vi "Configure_single_acquisition.vi"(8 "error in (no error)":errorcluster, 11 "Initialize_card in":refnum<class "Initialize_card.lvclass">) -> (0 "error out":errorcluster, 3 "Initialize_card out":refnum<class "Initialize_card.lvclass">)   [LabVIEW 2015, in "Initialize_card.lvclass"]
uses:
  Initialize_card.lvclass
panel:
  in  "Extended Options (0)":i32
  in  "Invert Clock (f)":bool
  out "Error Code":i32
  in  "Segment Count (1)":u32=1
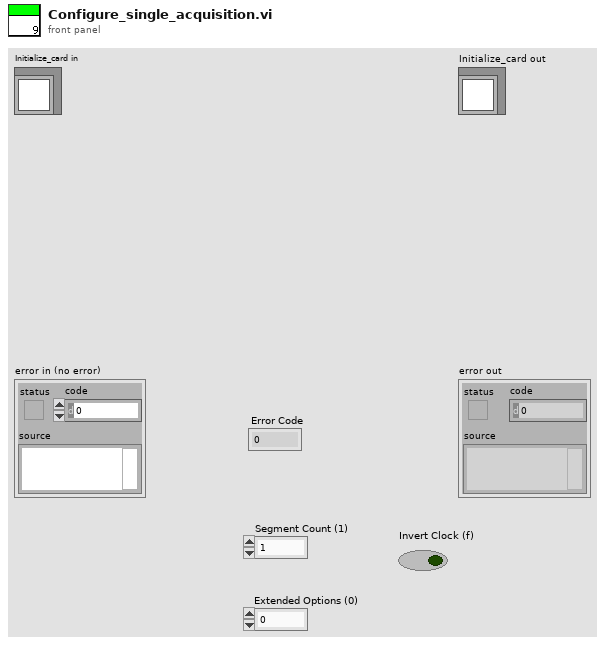
[diagram p1: front panel]
types:
  T1 = cluster{"Sample Rate":dbl, "Clock mode":enum16{"Internal", "External", "Reference"}, "Mode":u16, "Depth":dbl, "Segment Size":dbl, "Trigger Timeout":dbl, "Trigger Holdoff":dbl, "Trigger Delay":dbl}
  T2 = cluster{"Handle":u32, "Sample size":u32, "Resolution":i32, "Offset":i32, "Channels":u32, "Boards":u32}
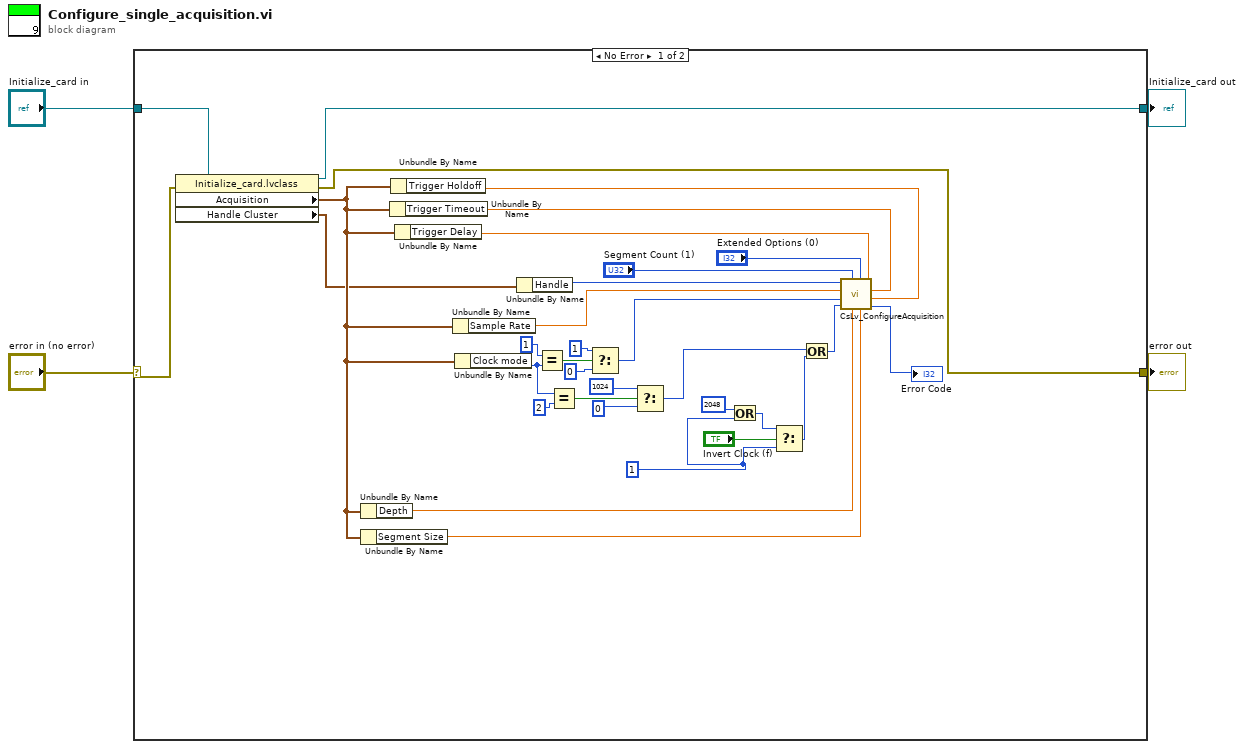
[diagram p0: block diagram]
diagram:
  n1 = case shown="No Error" "error in (no error)" {
    selector: "error in (no error)" -> [w9 w39]
    tunnel: [w8 w39] -> w3
    tunnel: [w10 w38] -> w1
    tunnel: "Initialize_card in" -> [w11 w38]
    frame No Error {
      w6 = 1 ("y")
      n2 = property class="Initialize_card.lvclass"(reference=w11, error in=w9) -> (reference out=w10:refnum<class "Initialize_card.lvclass">, error out=w8:errorcluster, "Acquisition"=w7:T1, "Handle Cluster"=w5:T2)
      n3 = Unbundle By Name(w7) -> ("Depth"=w33:dbl)
      n4 = Unbundle By Name(w7) -> ("Segment Size"=w25:dbl)
      n5 = Unbundle By Name(w7) -> ("Trigger Timeout"=w31:dbl)
      n6 = Unbundle By Name(w7) -> ("Trigger Holdoff"=w30:dbl)
      n7 = Unbundle By Name(w7) -> ("Trigger Delay"=w32:dbl)
      n8 = Unbundle By Name(w7) -> ("Sample Rate"=w34:dbl)
      n9 = Unbundle By Name(w7) -> ("Clock mode"=w19:enum16{"Internal", "External", "Reference"})
      n10 = Unbundle By Name(w5) -> ("Handle"=w37:u32)
      n11 = Equal?(x=1, y=w19) -> (x = y?=w24:bool)
      n12 = Equal?(x=w19, y=2) -> (x = y?=w17:bool)
      n13 = Select(t=1, s=w24, f=0) -> (s? t:f=w23:i32)
      n14 = Select(t=1024, s=w17, f=0) -> (s? t:f=w12:i32)
      n15 = Or(x=2048, y=w6) -> (x .or. y?=w27:i32)
      n16 = Select(t=w27, s="Invert Clock (f)", f=w6) -> (s? t:f=w13:i32)
      n17 = Or(x=w12, y=w13) -> (x .or. y?=w14:i32)
      n18 = call <userlib>:"CsLv_ConfigureAcquisition.vi"("Trigger Holdoff (0)"=w30, "Trigger Timeout (10000000)"=w31, "Trigger Delay (0)"=w32, "Segment Size (8192)"=w25, "Extended Options (0)"="Extended Options (0)", "Depth (8192)"=w33, "Segment Count (1)"="Segment Count (1)", "Mode (2)"=w14, "External Clock (0)"=w23, "Sample Rate (100000000)"=w34, "Handle"=w37) -> ("Error Code"=→"Error Code":i32)
    }
    frame Error {
    }
  }
  "error out" <- w3
  "Initialize_card out" <- w1
